vi "BRig_RT__Case_Exp__State_initTrial__LC_Select.vi"(6 "input_arrTrig":bool[](array[boolean]), 8 "input_dataTrial":u16[][](array[numeric]), 9 "input_dataExp":u16[](array[numeric]), 10 "input_dataLC":u16[](array[numeric]), 11 "input_dataCurrent":u16[](array[numeric])) -> (0 "output_dataTrial":u16[][](array[numeric]), 3 "output_dataCurrent":u16[](array[numeric]), 4 "output_arrTrig":bool[](array[boolean]))   [LabVIEW 2014]
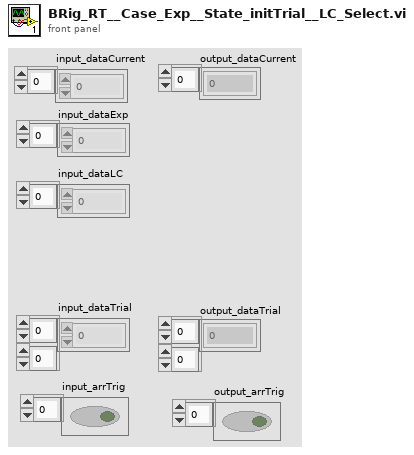
[diagram p1: front panel]
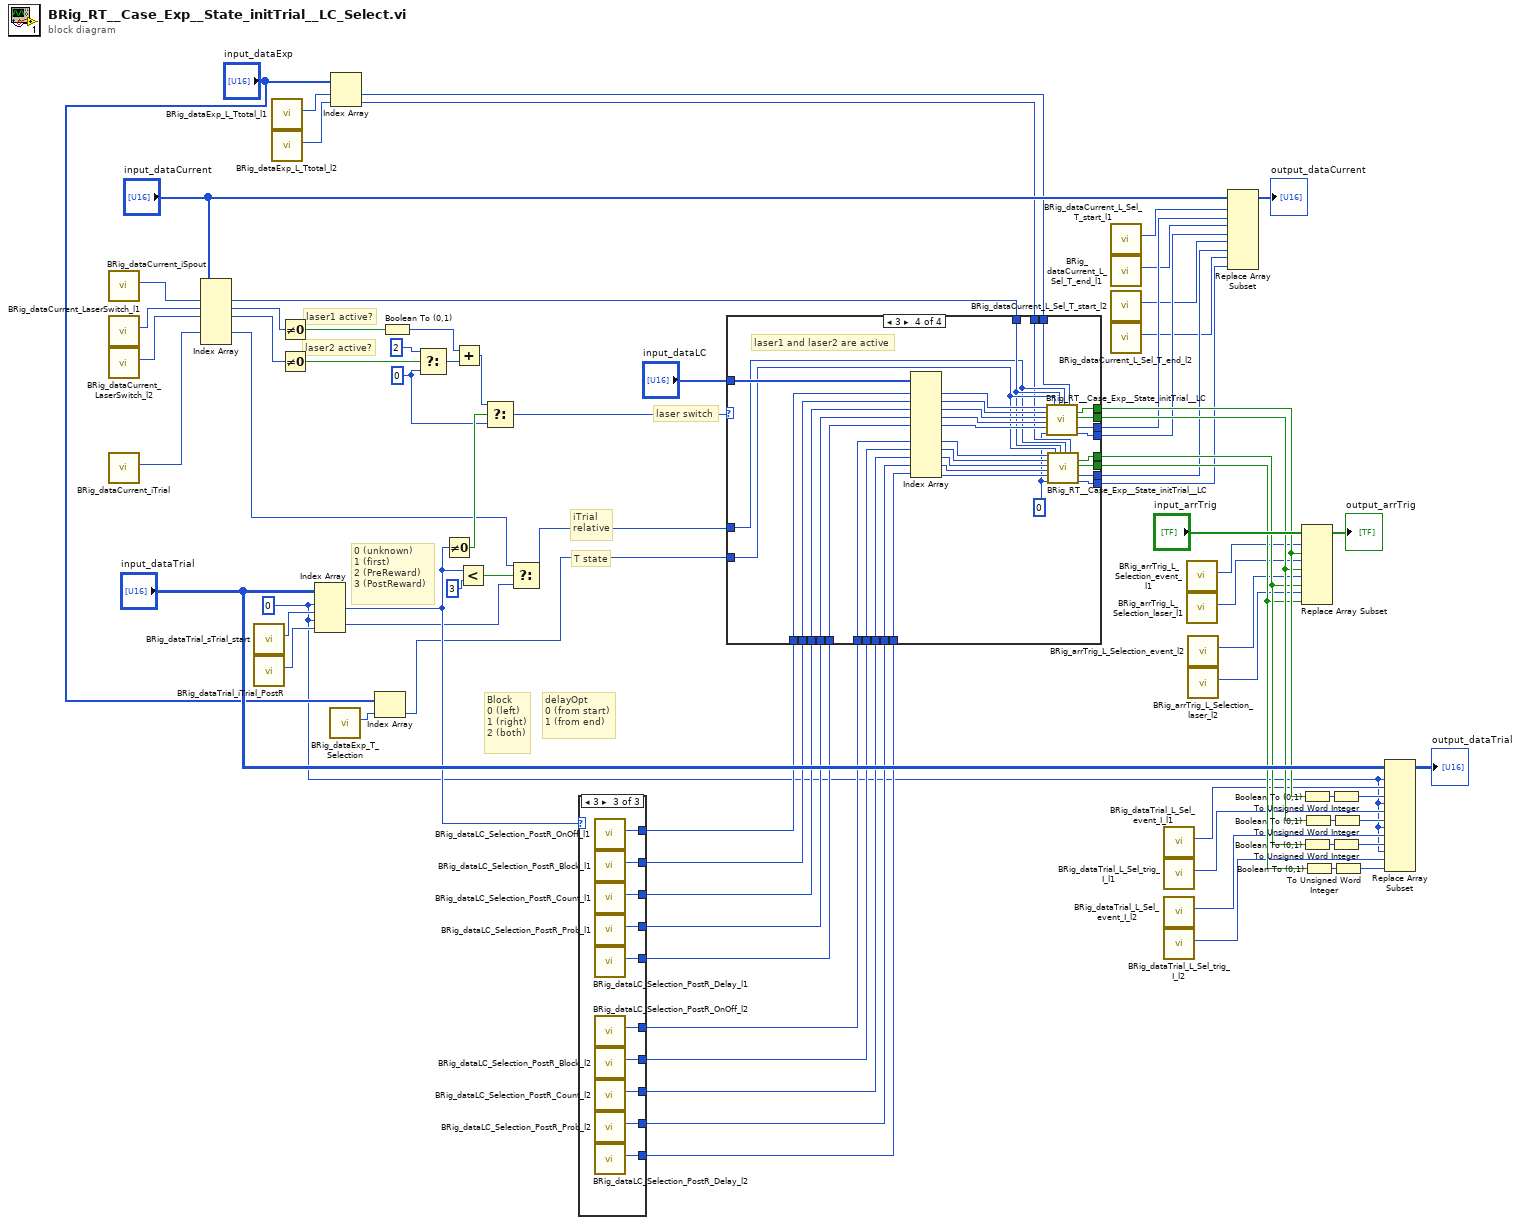
[diagram p0: block diagram]
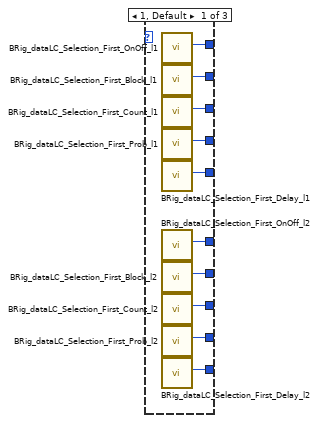
[diagram p2: hidden frame]
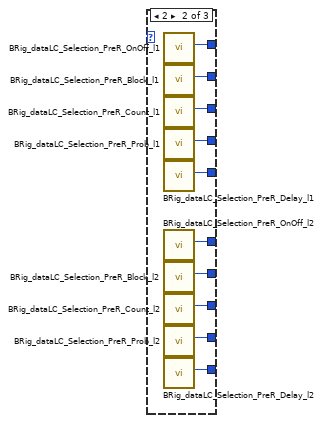
[diagram p3: hidden frame]
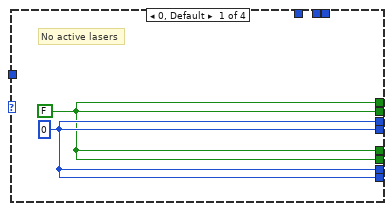
[diagram p4: hidden frame]
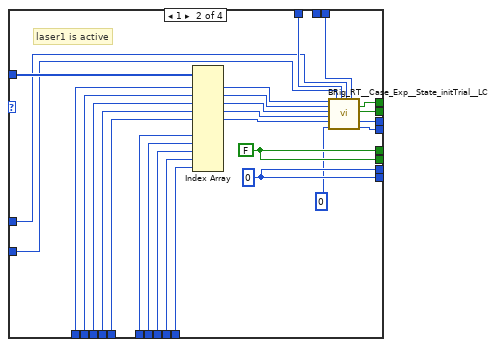
[diagram p5: hidden frame]
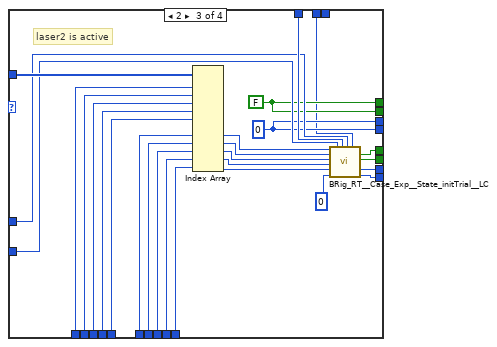
[diagram p6: hidden frame]
diagram:
  w1 = 0
  w66 = i16 0 ("f")
  # "iTrial\nrelative"
  # "laser switch"
  # "T state"
  # "delayOpt\n0 (from start)\n1 (from end)"
  # "Block\n0 (left)\n1 (right)\n2 (both)"
  # "0 (unknown)\n1 (first)\n2 (PreReward)\n3 (PostReward)"
  # "laser2 active?"
  # "laser1 active?"
  n1 = call "BRig_dataCurrent_iSpout.vi"() -> ("output_iSpout"=w62:i32)  [unwired: 11 in]
  n2 = call "BRig_dataCurrent_LaserSwitch_l1.vi"() -> ("output_LaserSwitch_l1"=w77:i32)  [unwired: 11 in]
  n3 = call "BRig_dataCurrent_LaserSwitch_l2.vi"() -> ("output_LaserSwitch_l2"=w76:i32)  [unwired: 11 in]
  n4 = call "BRig_dataCurrent_iTrial.vi"() -> ("output_iTrial"=w8:i32)  [unwired: 11 in]
  n5 = Index Array(array="input_dataCurrent", index #1=w62, index #2=w77, index #3=w76, index #5=w8) -> (element #1=w61:u16, element #2=w75:u16, element #3=w74:u16, element #5=w6:u16)  [unwired: 2 in, 2 out]
  n6 = call "BRig_dataTrial_sTrial_start.vi"() -> ("output_sTrial_start"=w73:i32)  [unwired: 11 in]
  n7 = call "BRig_dataTrial_iTrial_PostR.vi"() -> ("output_iTrial_PostR"=w4:i32)  [unwired: 11 in]
  n8 = call "BRig_dataExp_L_Ttotal_l1.vi"() -> ("output_L_Ttotal_l1"=w25:i32)  [unwired: 11 in]
  n9 = call "BRig_dataExp_L_Ttotal_l2.vi"() -> ("output_L_Ttotal_l2"=w26:i32)  [unwired: 11 in]
  n10 = Not Equal To 0?(x=w75) -> (x != 0?=w72:bool)
  n11 = Not Equal To 0?(x=w74) -> (x != 0?=w71:bool)
  n12 = Index Array(array="input_dataTrial", index (row) #1=w1, index (col) #1=w73, index (row) #2=w1, index (col) #2=w4) -> (element #1=w38:u16, element #2=w3:u16)
  n13 = call "BRig_dataExp_T_Selection.vi"() -> ("output_T_Selection"=w22:i32)  [unwired: 11 in]
  n14 = Index Array(array="input_dataExp", index #1=w25, index #2=w26) -> (element #1=w23:u16, element #2=w24:u16)
  n15 = Index Array(array="input_dataExp", index=w22) -> (element=w2:u16)
  n16 = Boolean To (0,1)(Boolean=w72) -> (0, 1=w68:i16)
  n17 = Select(t=i16 2, s=w71, f=w66) -> (s? t:f=w69:i16)
  n18 = Not Equal To 0?(x=w38) -> (x != 0?=w67:bool)
  n19 = Add(x=w68, y=w69) -> (x+y=w65:i16)
  n20 = Less?(x=w38, y=u16 3) -> (x < y?=w7:bool)
  n21 = Select(t=w65, s=w67, f=w66) -> (s? t:f=w64:i16)
  n22 = Select(t=w6, s=w7, f=w3) -> (s? t:f=w5:u16)
  n23 = case shown="3" w38 {
    tunnel: [w87 w97 w107] -> w37
    tunnel: [w80 w95 w105] -> w36
    tunnel: [w81 w94 w104] -> w35
    tunnel: [w82 w93 w103] -> w34
    tunnel: [w83 w92 w102] -> w33
    tunnel: [w86 w96 w106] -> w32
    tunnel: [w84 w91 w101] -> w31
    tunnel: [w85 w90 w100] -> w30
    tunnel: [w78 w89 w99] -> w29
    tunnel: [w79 w88 w98] -> w28
    frame 1, Default {
      n24 = call "BRig_dataLC_Selection_First_OnOff_l1.vi"() -> ("output_Selection_First_OnOff"=w87:i32)  [unwired: 11 in]
      n25 = call "BRig_dataLC_Selection_First_Block_l1.vi"() -> ("output_Selection_First_Block"=w80:i32)  [unwired: 11 in]
      n26 = call "BRig_dataLC_Selection_First_Count_l1.vi"() -> ("output_Selection_First_Count"=w81:i32)  [unwired: 11 in]
      n27 = call "BRig_dataLC_Selection_First_Prob_l1.vi"() -> ("output_Selection_First_Prob"=w82:i32)  [unwired: 11 in]
      n28 = call "BRig_dataLC_Selection_First_Delay_l1.vi"() -> ("output_Selection_First_Delay"=w83:i32)  [unwired: 11 in]
      n29 = call "BRig_dataLC_Selection_First_OnOff_l2.vi"() -> ("output_Selection_First_OnOff_l2"=w86:i32)  [unwired: 11 in]
      n30 = call "BRig_dataLC_Selection_First_Block_l2.vi"() -> ("output_Selection_First_Block_l2"=w84:i32)  [unwired: 11 in]
      n31 = call "BRig_dataLC_Selection_First_Count_l2.vi"() -> ("output_Selection_First_Count_l2"=w85:i32)  [unwired: 11 in]
      n32 = call "BRig_dataLC_Selection_First_Prob_l2.vi"() -> ("output_Selection_First_Prob_l2"=w78:i32)  [unwired: 11 in]
      n33 = call "BRig_dataLC_Selection_First_Delay_l2.vi"() -> ("output_Selection_First_Delay_l2"=w79:i32)  [unwired: 11 in]
    }
    frame 2 {
      n34 = call "BRig_dataLC_Selection_PreR_OnOff_l1.vi"() -> ("output_Selection_PreR_OnOff"=w97:i32)  [unwired: 11 in]
      n35 = call "BRig_dataLC_Selection_PreR_Block_l1.vi"() -> ("output_Selection_PreR_Block"=w95:i32)  [unwired: 11 in]
      n36 = call "BRig_dataLC_Selection_PreR_Count_l1.vi"() -> ("output_Selection_PreR_Count"=w94:i32)  [unwired: 11 in]
      n37 = call "BRig_dataLC_Selection_PreR_Prob_l1.vi"() -> ("output_Selection_PreR_Prob"=w93:i32)  [unwired: 11 in]
      n38 = call "BRig_dataLC_Selection_PreR_Delay_l1.vi"() -> ("output_Selection_PreR_Delay"=w92:i32)  [unwired: 11 in]
      n39 = call "BRig_dataLC_Selection_PreR_OnOff_l2.vi"() -> ("output_Selection_PreR_OnOff_l2"=w96:i32)  [unwired: 11 in]
      n40 = call "BRig_dataLC_Selection_PreR_Block_l2.vi"() -> ("output_Selection_PreR_Block_l2"=w91:i32)  [unwired: 11 in]
      n41 = call "BRig_dataLC_Selection_PreR_Count_l2.vi"() -> ("output_Selection_PreR_Count_l2"=w90:i32)  [unwired: 11 in]
      n42 = call "BRig_dataLC_Selection_PreR_Prob_l2.vi"() -> ("output_Selection_PreR_Prob_l2"=w89:i32)  [unwired: 11 in]
      n43 = call "BRig_dataLC_Selection_PreR_Delay_l2.vi"() -> ("output_Selection_PreR_Delay_l2"=w88:i32)  [unwired: 11 in]
    }
    frame 3 {
      n44 = call "BRig_dataLC_Selection_PostR_OnOff_l1.vi"() -> ("output_Selection_PostR_OnOff"=w107:i32)  [unwired: 11 in]
      n45 = call "BRig_dataLC_Selection_PostR_Block_l1.vi"() -> ("output_Selection_PostR_Block"=w105:i32)  [unwired: 11 in]
      n46 = call "BRig_dataLC_Selection_PostR_Count_l1.vi"() -> ("output_Selection_PostR_Count"=w104:i32)  [unwired: 11 in]
      n47 = call "BRig_dataLC_Selection_PostR_Prob_l1.vi"() -> ("output_Selection_PostR_Prob"=w103:i32)  [unwired: 11 in]
      n48 = call "BRig_dataLC_Selection_PostR_Delay_l1.vi"() -> ("output_Selection_PostR_Delay"=w102:i32)  [unwired: 11 in]
      n49 = call "BRig_dataLC_Selection_PostR_OnOff_l2.vi"() -> ("output_Selection_PostR_OnOff_l2"=w106:i32)  [unwired: 11 in]
      n50 = call "BRig_dataLC_Selection_PostR_Block_l2.vi"() -> ("output_Selection_PostR_Block_l2"=w101:i32)  [unwired: 11 in]
      n51 = call "BRig_dataLC_Selection_PostR_Count_l2.vi"() -> ("output_Selection_PostR_Count_l2"=w100:i32)  [unwired: 11 in]
      n52 = call "BRig_dataLC_Selection_PostR_Prob_l2.vi"() -> ("output_Selection_PostR_Prob_l2"=w99:i32)  [unwired: 11 in]
      n53 = call "BRig_dataLC_Selection_PostR_Delay_l2.vi"() -> ("output_Selection_PostR_Delay_l2"=w98:i32)  [unwired: 11 in]
    }
  }
  n54 = case shown="3" w64 {
    tunnel: "input_dataLC" -> [_ w136 w163 w198]
    tunnel: w61 -> [_ w129 w156 w186]
    tunnel: w2 -> [_ w130 w157 w187]
    tunnel: w5 -> [_ w128 w155 w185]
    tunnel: [w108 w127 w140 w184] -> w52
    tunnel: [w108 w126 w140 w183] -> w49
    tunnel: [w109 w125 w139 w182] -> w42
    tunnel: [w109 w124 w139 w181] -> w41
    tunnel: [w108 w113 w154 w180] -> w45
    tunnel: [w109 w112 w153 w179] -> w40
    tunnel: [w108 w113 w152 w178] -> w47
    tunnel: [w109 w112 w151 w177] -> w39
    tunnel: w37 -> [_ w123 w150 w176]
    tunnel: w36 -> [_ w122 w149 w175]
    tunnel: w35 -> [_ w121 w148 w174]
    tunnel: w34 -> [_ w120 w147 w173]
    tunnel: w33 -> [_ w119 w146 w172]
    tunnel: w32 -> [_ w118 w145 w171]
    tunnel: w31 -> [_ w117 w144 w170]
    tunnel: w30 -> [_ w116 w143 w169]
    tunnel: w29 -> [_ w115 w142 w168]
    tunnel: w28 -> [_ w114 w141 w167]
    tunnel: w24 -> [_ _ w138 w166]
    tunnel: w23 -> [_ w111 _ w165]
    frame 0, Default {
      w109 = u16 0
      w108 = FALSE
      # "No active lasers"
    }
    frame 1 {
      w112 = u16 0
      w113 = FALSE
      # "laser1 is active"
      n55 = Index Array(array=w136, index #1=w123, index #2=w122, index #3=w121, index #4=w120, index #5=w119, index #7=w118, index #8=w117, index #9=w116, index #10=w115, index #11=w114) -> (element #1=w135:u16, element #2=w134:u16, element #3=w133:u16, element #4=w132:u16, element #5=w131:u16)  [unwired: 1 in, 6 out]
      n56 = call "BRig_RT__Case_Exp__State_initTrial__LC.vi"("input_L_OnOff"=w135, "input_L_Block"=w134, "input_L_Count"=w133, "input_L_Prob"=w132, "input_L_Tdelay"=w131, "input_L_delayOpt"=u16 0, "input_T_state"=w130, "input_iSpout"=w129, "input_iTrial_relative"=w128, "input_L_T"=w111) -> ("output_LC_Event"=w127:bool, "output_LC_Laser"=w126:bool, "output_L_Tstart"=w125:u16, "output_L_Tend"=w124:u16)  [unwired: 6 in]
    }
    frame 2 {
      w139 = u16 0
      w140 = FALSE
      # "laser2 is active"
      n57 = Index Array(array=w163, index #1=w150, index #2=w149, index #3=w148, index #4=w147, index #5=w146, index #7=w145, index #8=w144, index #9=w143, index #10=w142, index #11=w141) -> (element #7=w158:u16, element #8=w159:u16, element #9=w160:u16, element #10=w161:u16, element #11=w162:u16)  [unwired: 1 in, 6 out]
      n58 = call "BRig_RT__Case_Exp__State_initTrial__LC.vi"("input_L_OnOff"=w158, "input_L_Block"=w159, "input_L_Count"=w160, "input_L_Prob"=w161, "input_L_Tdelay"=w162, "input_L_delayOpt"=u16 0, "input_T_state"=w157, "input_iSpout"=w156, "input_iTrial_relative"=w155, "input_L_T"=w138) -> ("output_LC_Event"=w152:bool, "output_LC_Laser"=w154:bool, "output_L_Tstart"=w153:u16, "output_L_Tend"=w151:u16)  [unwired: 6 in]
    }
    frame 3 {
      w164 = u16 0 ("input_L_delayOpt")
      # "laser1 and laser2 are active"
      n59 = Index Array(array=w198, index #1=w176, index #2=w175, index #3=w174, index #4=w173, index #5=w172, index #7=w171, index #8=w170, index #9=w169, index #10=w168, index #11=w167) -> (element #1=w197:u16, element #2=w196:u16, element #3=w195:u16, element #4=w194:u16, element #5=w193:u16, element #7=w188:u16, element #8=w189:u16, element #9=w190:u16, element #10=w191:u16, element #11=w192:u16)  [unwired: 1 in, 1 out]
      n60 = call "BRig_RT__Case_Exp__State_initTrial__LC.vi"("input_L_OnOff"=w197, "input_L_Block"=w196, "input_L_Count"=w195, "input_L_Prob"=w194, "input_L_Tdelay"=w193, "input_L_delayOpt"=w164, "input_T_state"=w187, "input_iSpout"=w186, "input_iTrial_relative"=w185, "input_L_T"=w165) -> ("output_LC_Event"=w184:bool, "output_LC_Laser"=w183:bool, "output_L_Tstart"=w182:u16, "output_L_Tend"=w181:u16)  [unwired: 6 in]
      n61 = call "BRig_RT__Case_Exp__State_initTrial__LC.vi"("input_L_OnOff"=w188, "input_L_Block"=w189, "input_L_Count"=w190, "input_L_Prob"=w191, "input_L_Tdelay"=w192, "input_L_delayOpt"=w164, "input_T_state"=w187, "input_iSpout"=w186, "input_iTrial_relative"=w185, "input_L_T"=w166) -> ("output_LC_Event"=w178:bool, "output_LC_Laser"=w180:bool, "output_L_Tstart"=w179:u16, "output_L_Tend"=w177:u16)  [unwired: 6 in]
    }
  }
  n62 = call "BRig_dataCurrent_L_Sel_T_start_l1.vi"() -> ("output_L_Sel_T_start_l1"=w20:i32)  [unwired: 11 in]
  n63 = call "BRig_dataCurrent_L_Sel_T_end_l1.vi"() -> ("output_L_Sel_T_end_l1"=w19:i32)  [unwired: 11 in]
  n64 = call "BRig_dataCurrent_L_Sel_T_start_l2.vi"() -> ("output_L_Sel_T_start_l2"=w18:i32)  [unwired: 11 in]
  n65 = call "BRig_dataCurrent_L_Sel_T_end_l2.vi"() -> ("output_L_Sel_T_end_l2"=w17:i32)  [unwired: 11 in]
  n66 = call "BRig_dataTrial_L_Sel_event_I_l1.vi"() -> ("output_L_Sel_event_I_l1"=w16:i32)  [unwired: 11 in]
  n67 = call "BRig_dataTrial_L_Sel_trig_I_l1.vi"() -> ("output_L_Sel_trig_I_l1"=w15:i32)  [unwired: 11 in]
  n68 = call "BRig_dataTrial_L_Sel_event_I_l2.vi"() -> ("output_L_Sel_event_I_l2"=w14:i32)  [unwired: 11 in]
  n69 = call "BRig_dataTrial_L_Sel_trig_I_l2.vi"() -> ("output_L_Sel_trig_I_l2"=w13:i32)  [unwired: 11 in]
  n70 = call "BRig_arrTrig_L_Selection_event_l1.vi"() -> ("output_L_Sel_event_l1"=w12:i32)  [unwired: 11 in]
  n71 = call "BRig_arrTrig_L_Selection_laser_l1.vi"() -> ("output_L_Sel_laserTrig_l1"=w11:i32)  [unwired: 11 in]
  n72 = call "BRig_arrTrig_L_Selection_event_l2.vi"() -> ("output_L_Sel_event_l2"=w10:i32)  [unwired: 11 in]
  n73 = call "BRig_arrTrig_L_Selection_laser_l2.vi"() -> ("output_L_Sel_laserTrig_l2"=w9:i32)  [unwired: 11 in]
  n74 = Replace Array Subset(array="input_dataCurrent", new element #1=w42, index #1=w20, new element #2=w41, index #2=w19, new element #3=w40, index #3=w18, new element #4=w39, index #4=w17) -> (→"output_dataCurrent":u16[])
  n75 = Replace Array Subset(array="input_arrTrig", new element #1=w52, index #1=w12, new element #2=w49, index #2=w11, new element #3=w47, index #3=w10, new element #4=w45, index #4=w9) -> (→"output_arrTrig":bool[])
  n76 = Boolean To (0,1)(Boolean=w52) -> (0, 1=w57:i16)
  n77 = Boolean To (0,1)(Boolean=w47) -> (0, 1=w54:i16)
  n78 = Boolean To (0,1)(Boolean=w49) -> (0, 1=w56:i16)
  n79 = Boolean To (0,1)(Boolean=w45) -> (0, 1=w55:i16)
  n80 = To Unsigned Word Integer(number=w57) -> (unsigned 16bit integer=w51:u16)
  n81 = To Unsigned Word Integer(number=w54) -> (unsigned 16bit integer=w48:u16)
  n82 = To Unsigned Word Integer(number=w56) -> (unsigned 16bit integer=w50:u16)
  n83 = To Unsigned Word Integer(number=w55) -> (unsigned 16bit integer=w46:u16)
  n84 = Replace Array Subset(array="input_dataTrial", new element #1=w51, index (row) #1=w1, index (col) #1=w16, new element #2=w50, index (row) #2=w1, index (col) #2=w15, new element #3=w48, index (row) #3=w1, index (col) #3=w14, new element #4=w46, index (row) #4=w1, index (col) #4=w13) -> (→"output_dataTrial":u16[][])
